vi "Initialize XBox Controller.vi"(11 "XBox Device Index":i32) -> (0 "Rrror Out":errorcluster, 3 "Device ID":refnum<k1>, 5 "Joystick Info":T1(array[cluster]))   [LabVIEW 2011]
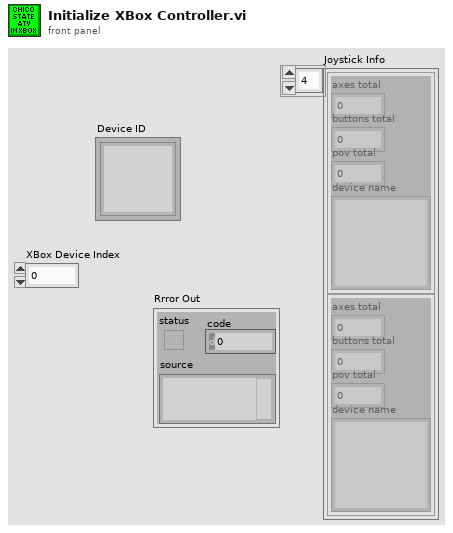
[diagram p1: front panel]
types:
  T1 = cluster{"axes total":u32, "buttons total":u32, "pov total":u32, "device name":string}[]
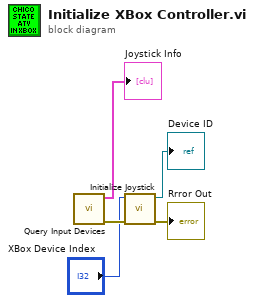
[diagram p0: block diagram]
diagram:
  n1 = call <vilib>:"Query Input Devices.vi"() -> ("error out"=w2:errorcluster, "joystick info"=→"Joystick Info":T1)  [unwired: 8 in, 2 out]
  n2 = call <vilib>:"Initialize Joystick.vi"("error in (no error)"=w2, "device index"="XBox Device Index") -> ("error out"=→"Rrror Out":errorcluster, "device ID"=→"Device ID":refnum<k1>)  [unwired: 8 in]
